vi "CIPeriod.vi"(8 "error in (no error)":errorcluster, 11 "reference":refnum<k24>) -> (0 "error out":errorcluster, 1 "StartingEdge":i32(ring) items=["Rising", "Falling"], 2 "MeasurementTime":dbl, 3 "reference out":refnum<k24>, 4 "Units":i32(ring) items=["Seconds", "Ticks"])   [LabVIEW 2009]
uses:
  C:/Program Files/National Instruments/LabVIEW 2009/vi.lib/ULx/ULx_LV.dll
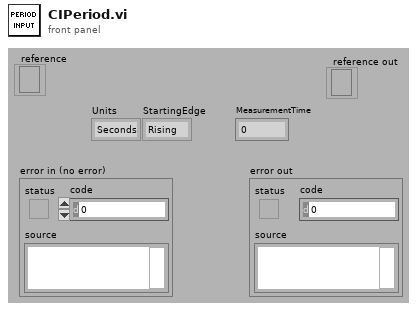
[diagram p1: front panel]
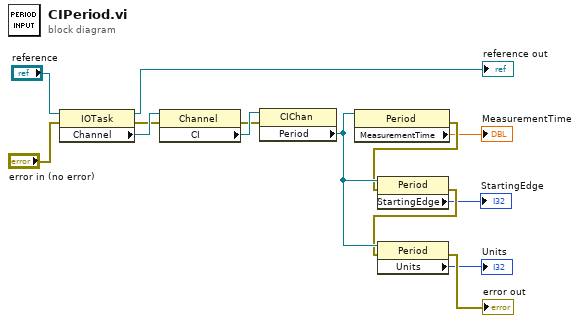
[diagram p0: block diagram]
diagram:
  n1 = property class="IOTask"(reference="reference", error in="error in (no error)") -> (reference out=→"reference out":refnum<k24>, error out=w9:errorcluster, "Channel"=w14:refnum<k24>)
  n2 = property class="Channel"(reference=w14, error in=w9) -> (error out=w8:errorcluster, "CI"=w13:refnum<k24>)  [unwired: 1 out]
  n3 = property class="CIChan"(reference=w13, error in=w8) -> ("Period"=w7:refnum<k24>)  [unwired: 2 out]
  n4 = property class="Period"(reference=w7) -> (error out=w6:errorcluster, "MeasurementTime"=→"MeasurementTime":dbl)  [unwired: 1 in, 1 out]
  n5 = property class="Period"(reference=w7, error in=w6) -> (error out=w5:errorcluster, "StartingEdge"=→"StartingEdge":i32)  [unwired: 1 out]
  n6 = property class="Period"(reference=w7, error in=w5) -> (error out=→"error out":errorcluster, "Units"=→"Units":i32)  [unwired: 1 out]
